vi "Close.vi"(8 "error in (no error)":errorcluster, 11 "ZanClass in":refnum<class "ZanClass.lvclass">) -> (0 "error out":errorcluster, 3 "ZanClass out":refnum<class "ZanClass.lvclass">)   [LabVIEW 2019, in "ZanClass.lvclass"]
uses:
  ZanClass.lvclass
  LLB/zmotion/zaux/zauxdll.lvlib
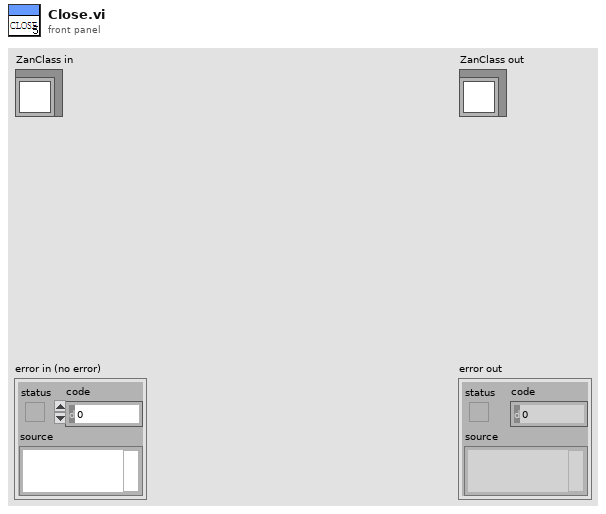
[diagram p1: front panel]
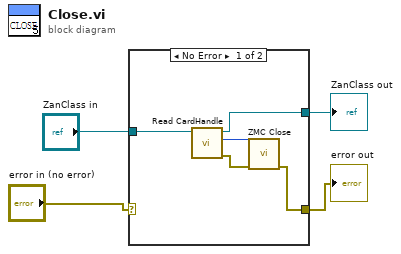
[diagram p0: block diagram]
diagram:
  n1 = case shown="No Error" "error in (no error)" {
    selector: "error in (no error)" -> [_ w10]
    tunnel: "ZanClass in" -> [w8 w11]
    tunnel: [w7 w11] -> w2
    tunnel: [w5 w10] -> w1
    frame No Error {
      n2 = call-dynamic "Read CardHandle.vi"("AxisCard in"=w8) -> ("error out"=w6:errorcluster, "CardHandle"=w9:i32, "AxisCard out"=w7:refnum<class "ZanClass.lvclass">)  [unwired: 8 in]
      n3 = call "ZMC Close.vi"("error in (no error)"=w6, "handle"=w9) -> ("error out"=w5:errorcluster)  [unwired: 7 in, 2 out]
    }
    frame Error {
    }
  }
  "error out" <- w1
  "ZanClass out" <- w2
